vi "Get Variables.vi"(8 "error in (no error)":errorcluster, 11 "Message Popup in":refnum<class "Statement.lvclass">) -> (0 "error out":errorcluster, 2 "Variables":variant, 3 "Message Popup out":refnum<class "Statement.lvclass">)   [LabVIEW 2019, in "Statement.lvclass"]
uses:
  Statement.lvclass
  Statement.lvclass/Statement.ctl
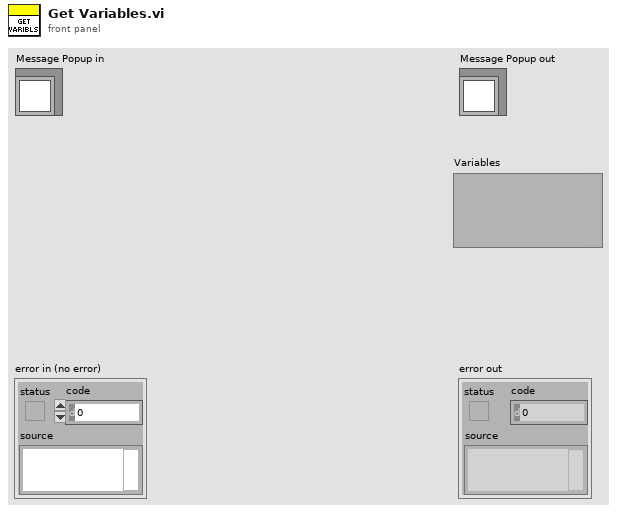
[diagram p1: front panel]
types:
  T1 = typedef "Statement.lvclass/Variables.ctl" = cluster{"leftoperand":string, "rightoperand":variant}
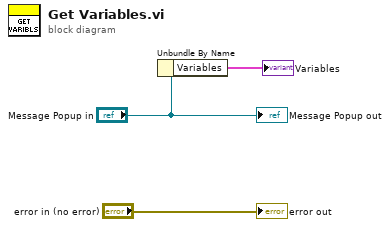
[diagram p0: block diagram]
diagram:
  n1 = Unbundle By Name("Message Popup in") -> ("Variables"=→"Variables":T1)
  "error out" <- "error in (no error)"
  "Message Popup out" <- "Message Popup in"
